vi "Get_filelist.vi"(8 "error in (no error)":errorcluster) -> (0 "error out":errorcluster, 2 "Files":string[](array[string]))   [LabVIEW 2024, in "FTPS.lvlib"]
uses:
  FTPS.lvlib
  <vilib>/FTP/ftp2.llb/FTP File Info.ctl
  <vilib>/FTP/NI_FTP.lvlib
  Launcher/Launcher_DTU.lvlib
panel:
  in  "address":string="169.254.73.100"
  out "dir list":T1[](array[typedef])
  out "reply string":string
  in  "ClusterSetting":T2={"password"="1234", "user"="ftpadmin", "remote path"="/River/ssl_config.csv", "host"="169.254.73.100"}
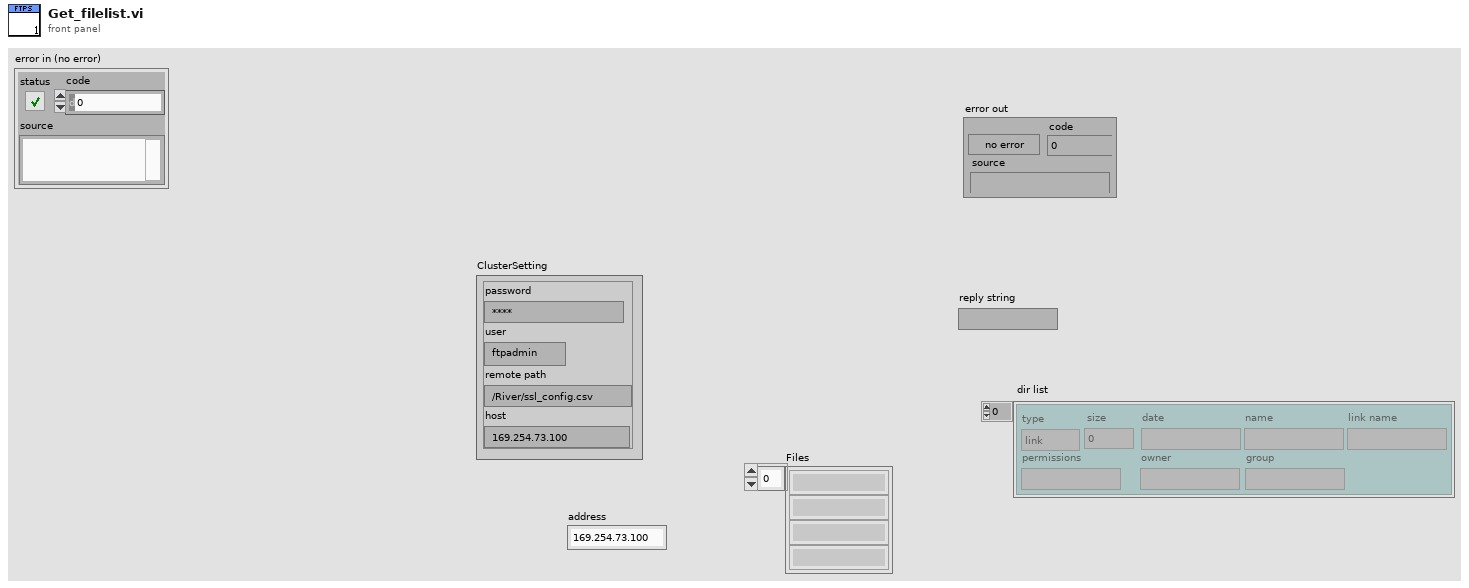
[diagram p1: front panel]
types:
  T1 = typedef "NI_FTP.lvlib/FTP File Info.ctl" = cluster{"type":enum16{"unknown", "file", "dir", "link"}, "permissions":string, "owner":string, "group":string, "size":i32, "date":string, "name":string, "link name":string}
  T2 = cluster{"password":string, "user":string, "remote path":string, "host":string}
  T3 = enum16{"Read", "Write", "All_sections", "All_values", "Remove key&section"}
  T4 = typedef "NI_FTP.lvlib/FTP Session.ctl" = refnum<k5>
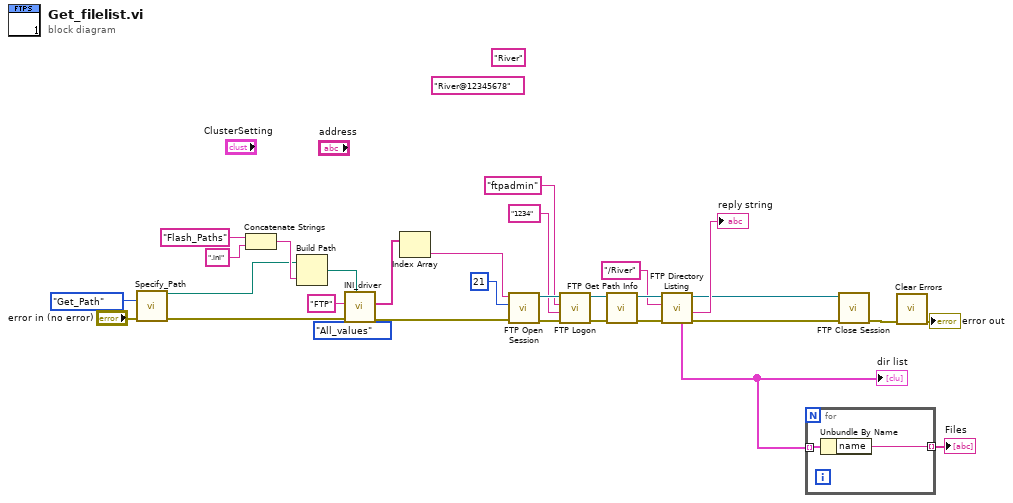
[diagram p0: block diagram]
diagram:
  (unwired) "River@12345678" ("password")
  (unwired) "River" ("user")
  n1 = call "Specify_Path.vi"("Path_Enum"=enum16{"Find_Path", "Get_Path"}."Get_Path", "error in (no error)"="error in (no error)") -> ("Configurations"=w8:path, "error out"=w12:errorcluster)  [unwired: 6 in, 6 out]
  n2 = Concatenate Strings("Flash_Paths" ("string"), ".ini" ("string")) -> (w14:string)
  n3 = Build Path(base path=w8, name or relative path=w14) -> (appended path=w13:path)
  n4 = call "INI_driver.vi"("Enum"=T3."All_values", "instrument file path"=w13, "error in (no error)"=w12, "Section"="FTP") -> ("error out"=w5:errorcluster, "Values out"=w7:string[])  [unwired: 4 in, 2 out]
  n5 = Index Array(array=w7) -> (element=w6:string)  [unwired: 1 in]
  n6 = call <vilib>:"FTP Open Session.vi"("error in (no error)"=w5, "remote port (21)"=u16 21, "address"=w6) -> ("error out"=w28:errorcluster, "ftp session"=w29:T4)  [unwired: 5 in, 2 out]
  n7 = call <vilib>:"FTP Logon.vi"("error in (no error)"=w28, "password"="1234", "user"="ftpadmin", "ftp session"=w29) -> ("error out"=w25:errorcluster, "ftp session out"=w24:T4)  [unwired: 4 in, 2 out]
  n8 = call <vilib>:"FTP Get Path Info.vi"("error in (no error)"=w25, "ftp session"=w24) -> ("error out"=w23:errorcluster, "ftp session out"=w22:T4)  [unwired: 5 in, 3 out]
  n9 = call <vilib>:"FTP Directory Listing.vi"("error in (no error)"=w23, "directory path"="/River", "ftp session"=w22) -> ("error out"=w19:errorcluster, "reply string"=→"reply string":string, "ftp session out"=w18:T4, "dir list"=w17:T1[])  [unwired: 4 in, 1 out]
  "dir list" <- w17
  n10 = for {
    tunnel: w17 -> [w32] mode=indexing
    tunnel: [w31] -> w3 mode=indexing
    n11 = Unbundle By Name(w32) -> ("name"=w31:string)
  }
  "Files" <- w3
  n12 = call <vilib>:"FTP Close Session.vi"("error in (no error)"=w19, "ftp session"=w18) -> ("error out"=w2:errorcluster)  [unwired: 6 in, 3 out]
  n13 = call <vilib>:"Clear Errors.vi"("error in (no error)"=w2) -> ("error out"=→"error out":errorcluster)  [unwired: 5 in, 1 out]
